vi "Change_Enum.vi"() -> ()   [LabVIEW 2013]
uses:
  <vilib>/Utility/file.llb/Read From Spreadsheet File (string).vi
panel:
  out "output array":string[](array[string])
  in  "file path (dialog if empty)":path
  in  "Strings []":string[](array[string])=["This", "is", "after"]
  in  "target class":refnum<vi>
  in  "vi path":path=path "enum_target.vi"
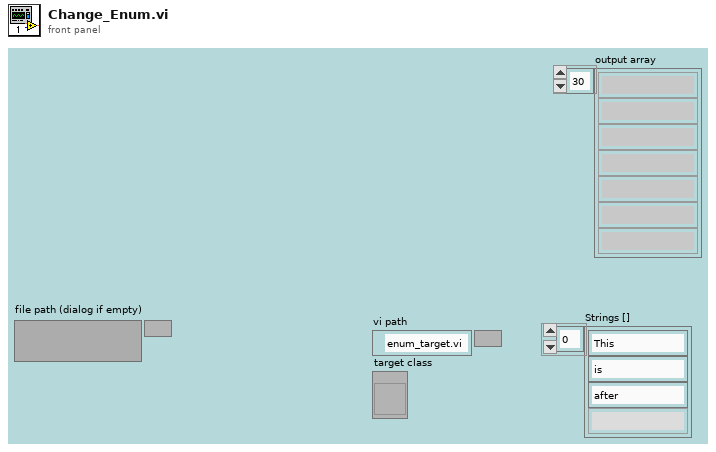
[diagram p1: front panel]
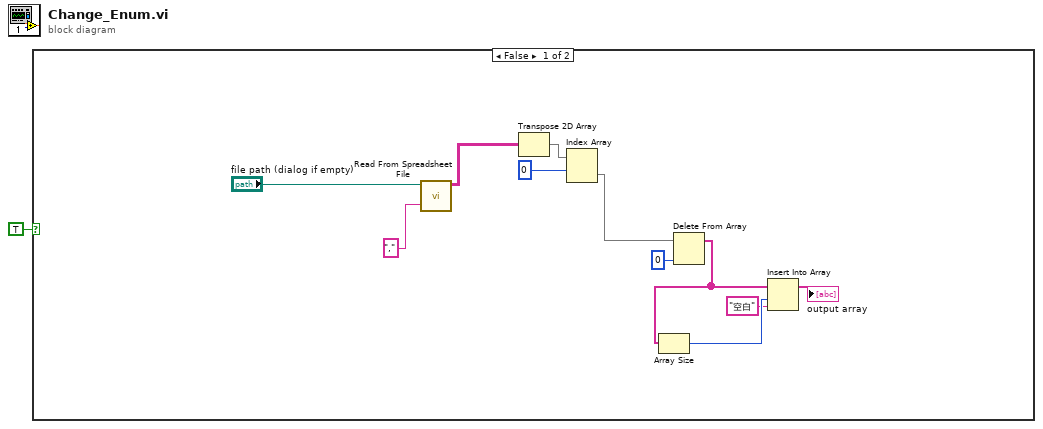
[diagram p0: block diagram]
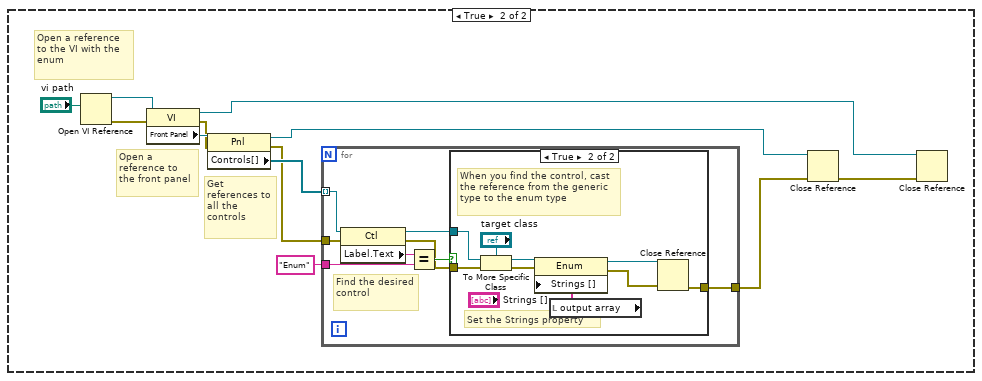
[diagram p2: hidden frame]
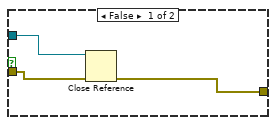
[diagram p3: hidden frame]
diagram:
  n1 = case shown="False" TRUE {
    frame False {
      n2 = call-poly <vilib>:"Read From Spreadsheet File.vi"("delimiter (\\t)"="," ("delimiter (\\t)"), "file path (dialog if empty)"="file path (dialog if empty)") -> ("all rows"=w10:string[][])  [unwired: 5 in, 4 out]
      n3 = Transpose 2D Array(2D array=w10) -> (transposed array=w9:string[][])
      n4 = Index Array(array=w9, index (row)=0) -> (element=w7:string[])  [unwired: 1 in]
      n5 = Delete From Array(array=w7, index=0) -> (array with subset deleted=w5:string[])  [unwired: 1 in, 1 out]
      n6 = Array Size(array=w5) -> (size(s)=w4:i32)
      n7 = Insert Into Array(array=w5, index=w4, new element="空白" ("new element/subarray")) -> (→"output array":string[])
    }
    frame True {
      # "Open a reference to the VI with the enum"
      # "Open a reference to the front panel"
      # "Get references to all the controls"
      n8 = Open VI Reference(vi path="vi path") -> (vi reference=w24:refnum<vi>, error out=w17:errorcluster)  [unwired: 5 in]
      n9 = property class="VI"(reference=w24, error in=w17) -> (reference out=w21:refnum<vi>, error out=w16:errorcluster, "Front Panel"=w23:refnum<vi>)
      n10 = property class="Pnl"(reference=w23, error in=w16) -> (reference out=w20:refnum<vi>, error out=w15:errorcluster, "Controls[]"=w19:refnum<vi>[])
      n11 = for {
        tunnel: w19 -> [w32] mode=indexing
        tunnel: "Enum" -> [w30]
        tunnel: w15 -> [w27]
        tunnel: [w25] -> w14
        # "Find the desired control"
        n12 = property class="Ctl"(reference=w32, error in=w27) -> (reference out=w28:refnum<vi>, error out=w26:errorcluster, "Label.Text"=w31:string)
        n13 = Equal?(x=w31, y=w30) -> (x = y?=w29:bool)
        n14 = case shown="True" w29 {
          tunnel: w28 -> [w35 w44]
          tunnel: w26 -> [w34 w40]
          tunnel: [w33 w37] -> w25
          frame False {
            n15 = Close Reference(reference=w35, error in (no error)=w34) -> (error out=w33:errorcluster)
          }
          frame True {
            # "Set the Strings property"
            # "When you find the control, cast the reference from the generic type to the enum type"
            n16 = To More Specific Class(target class="target class", reference=w44, error in=w40) -> (specific class reference=w42:refnum<vi>, error out=w39:errorcluster)
            n17 = local read "output array"() -> (w36:string[])
            n18 = property class="Enum"(reference=w42, error in=w39, "Strings []"=w36) -> (reference out=w41:refnum<vi>, error out=w38:errorcluster)
            n19 = Close Reference(reference=w41, error in (no error)=w38) -> (error out=w37:errorcluster)
          }
        }
      }
      n20 = Close Reference(reference=w20, error in (no error)=w14) -> (error out=w13:errorcluster)
      n21 = Close Reference(reference=w21, error in (no error)=w13) -> ()  [unwired: 1 out]
    }
  }
